vi "Initialise User login and application data.vi"(7 "mains application path":path, 8 "error in":errorcluster, 9 "Revision number":string, 10 "Strings []":string[](array[string]), 11 "Initialise cluster":T3={"wait value"=0.0, "Power supply"="COM1", "DMM"="COM1", "Arduino"="", "RS232 COM5"="", "RELAY BOARD"="COM1", "test sequence"=enum."Update Display", "Data folder path"=path "", "user account"="", "test sequence file name"="", "UI"=[], "DI"=[], "Skip test?"=[FALSE, FALSE, FALSE, FALSE, FALSE, FALSE, FALSE, FALSE, FALSE, FALSE, FALSE, FALSE, FALSE, FALSE, FALSE, FALSE, FALSE, FALSE, FALSE, FALSE, FALSE, FALSE, FALSE, FALSE, FALSE, FALSE, FALSE, FALSE, FALSE, FALSE, FALSE, FALSE], "Barcode"="", "DMM measuring state"=2, "T1"=[], "MCListbox Ref_in"=refnum, "RS232 COM6"="COM1", "mains application path"=path "", "sequence step #"=0, "Screening?"=FALSE, "Result?"=FALSE} {"DMM measuring state" items=["Voltage DC", "Voltage AC", "Current DC", "Current AC", "Resistance", "4-wire Resistance", "Diode", "Capacitance", "Temperature", "Continuity", "Frequency", "Period", "Voltage Ratio", "Voltage", "Current", "None"]; "DI"."Lower limit" format="%#_7f"}) -> (0 "error out":errorcluster, 1 "User name":i32 caption="Name(min 4 chars)", 2 "T1":string[][](array[string]), 3 "output cluster":T3={"wait value"=0.0, "Power supply"="COM1", "DMM"="COM1", "Arduino"="", "RS232 COM5"="", "RELAY BOARD"="COM1", "test sequence"=enum."Update Display", "Data folder path"=path "", "user account"="", "test sequence file name"="", "UI"=[], "DI"=[], "Skip test?"=[FALSE, FALSE, FALSE, FALSE, FALSE, FALSE, FALSE, FALSE, FALSE, FALSE, FALSE, FALSE, FALSE, FALSE, FALSE, FALSE, FALSE, FALSE, FALSE, FALSE, FALSE, FALSE, FALSE, FALSE, FALSE, FALSE, FALSE, FALSE, FALSE, FALSE, FALSE, FALSE], "Barcode"="", "DMM measuring state"=2, "T1"=[], "MCListbox Ref_in"=refnum, "RS232 COM6"="COM1", "mains application path"=path "", "sequence step #"=0, "Screening?"=FALSE, "Result?"=FALSE} {"DMM measuring state" items=["Voltage DC", "Voltage AC", "Current DC", "Current AC", "Resistance", "4-wire Resistance", "Diode", "Capacitance", "Temperature", "Continuity", "Frequency", "Period", "Voltage Ratio", "Voltage", "Current", "None"]; "DI"."Lower limit" format="%#_7f"}, 4 "Stop App?":bool, 5 "Varient&temp":T2, 6 "selected account name":string)   [LabVIEW 2021]
uses:
  controls/initialise cluster.ctl
  controls/developer_test sequence.ctl
  controls/test step description.ctl
  controls/test type selection.ctl
  controls/comparison selection.ctl
  controls/DMM measuring state.ctl
  controls/Control 1.ctl
  <vilib>/Utility/file.llb/Write Delimited Spreadsheet (string).vi
  <vilib>/Utility/file.llb/Read Delimited Spreadsheet (string).vi
panel:
  out "Data folder path":path
  out "test sequence file name":string
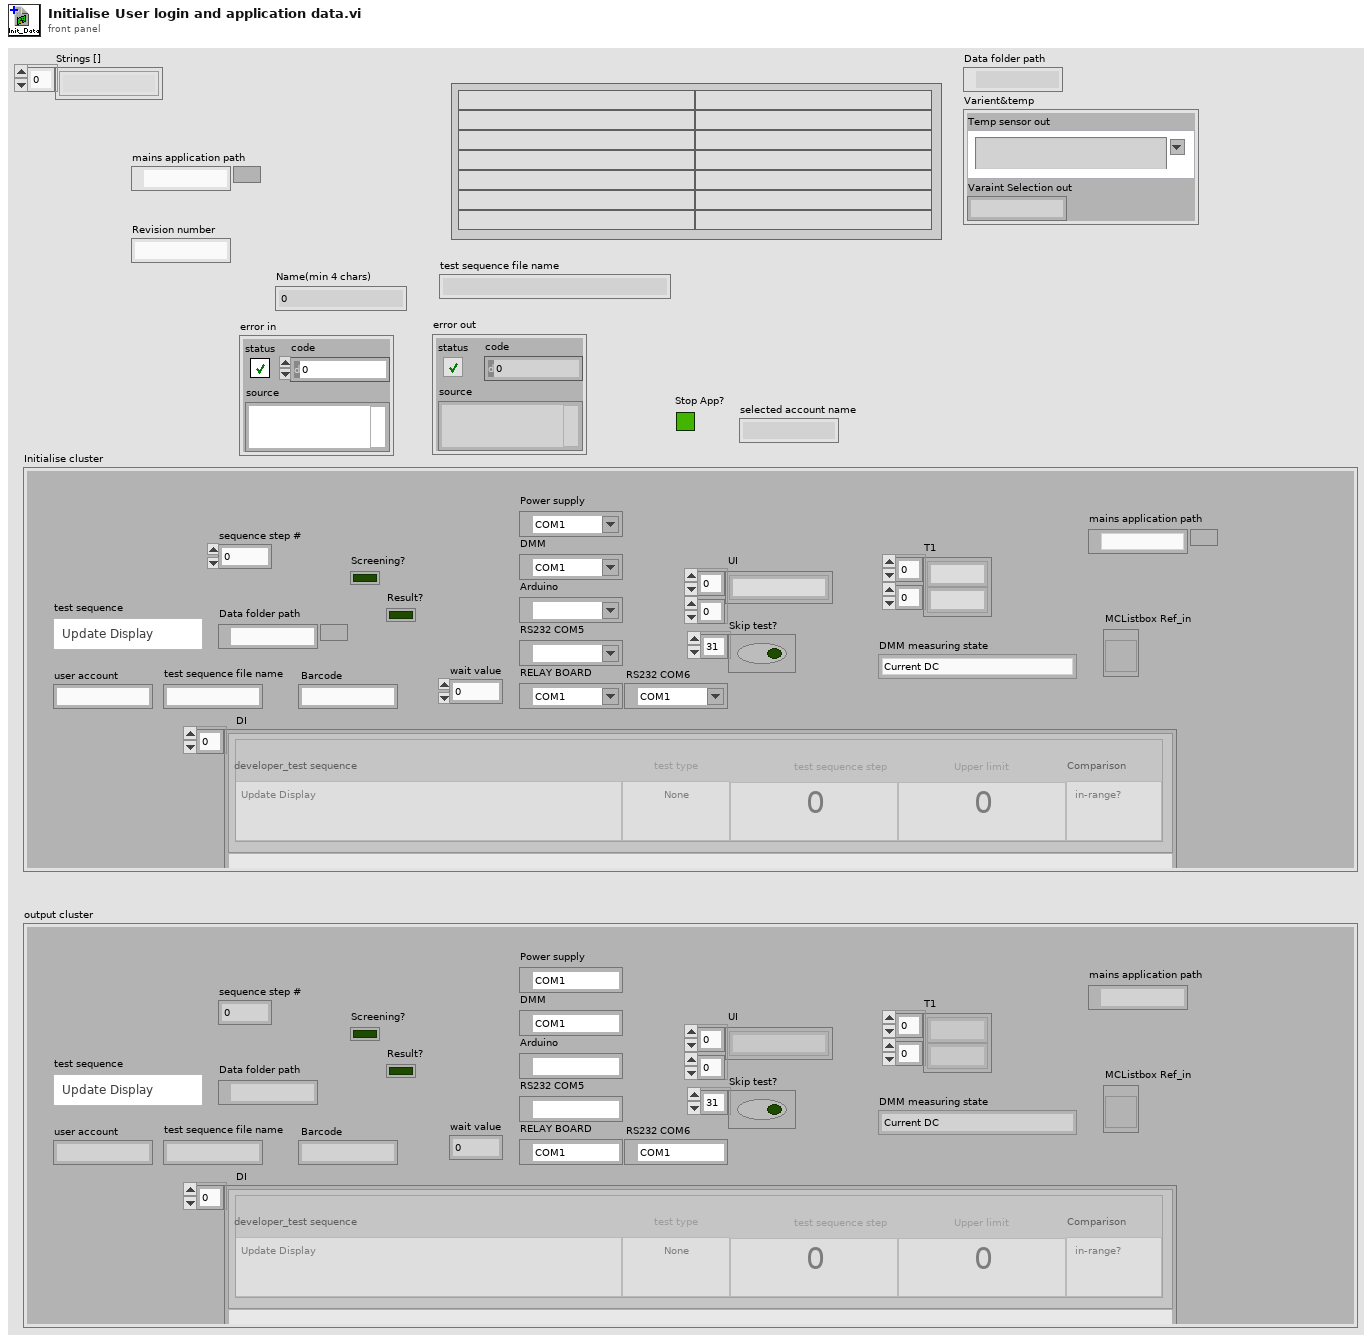
[diagram p1: front panel]
types:
  T1 = typedef "Control 1.ctl" = string
  T2 = cluster{"Temp sensor out":T1, "Varaint Selection out":string}
  T3 = typedef "initialise cluster.ctl" = cluster{"wait value":dbl, "Power supply":refnum<visa-resource-name>, "DMM":refnum<visa-resource-name>, "Arduino":refnum<visa-resource-name>, "RS232 COM5":refnum<visa-resource-name>, "RELAY BOARD":refnum<visa-resource-name>, "test sequence":T4, "Data folder path":path, "user account":string, "test sequence file name":string, "UI":string[][], "DI":T5[], "Skip test?":bool[], "Barcode":string, "DMM measuring state":T8, "T1":string[][], "MCListbox Ref_in":refnum<vi>, "RS232 COM6":refnum<visa-resource-name>, "mains application path":path, "sequence step #":u32, "Screening?":bool, "Result?":bool}
  T4 = typedef "developer_test sequence.ctl" = enum16{"Update Display", "User Login", "Admin", "Initialise", "Init Devices", "Idle State", "test steup", "Abort", "Start Display Board Auto Testing", "Scan Barcode", "Checking TEMP at Thermistor 1", "Checking TEMP at Thermistor 2", "Checking TEMP at Thermistor 3", "Checking TEMP at Thermistor 4 (Ambient)", "Voltage Health Check", "Hillpot connector check", "INSULATION Resistance test (Baseplate to Negative)", "INSULATION Resistance test (Baseplate to Positive)", "Voltage helath check before weld resistance", "Current contactor check", "WELD Resistance Test", "Stop Display Board Auto Testing", "All Pass", "Fail", "Report", "Error", "Confirm Quit", "Exit"}
  T5 = typedef "test step description.ctl" = cluster{"test type":T6, "developer_test sequence":T4, "Lower limit":dbl, "Upper limit":dbl, "Comparison":T7}
  T6 = typedef "test type selection.ctl" = enum16{"None", "Voltage", "Voltage?", "Current", "Current?", "Output", "Program"}
  T7 = typedef "comparison selection.ctl" = enum16{"None", "in-range?", "less than?", "greater than?", "equal to?", "not equal to?", "less or equal to?", "greater or equal to?"}
  T8 = typedef "DMM measuring state.ctl" = u16
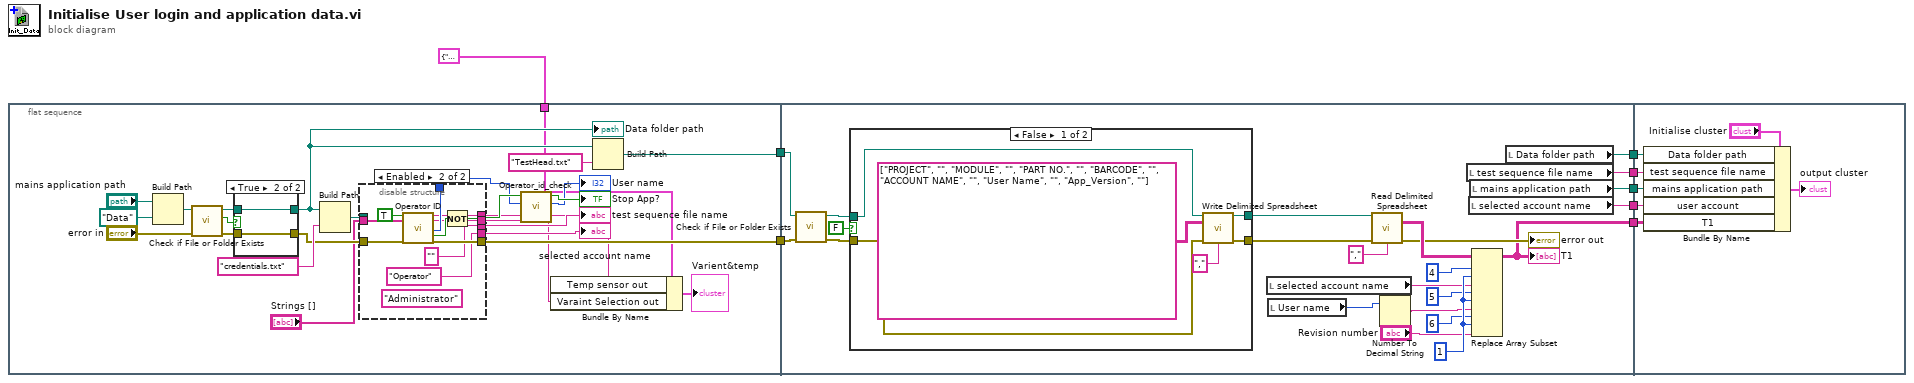
[diagram p0: block diagram]
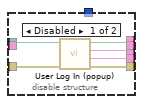
[diagram p2: hidden frame]
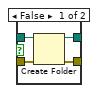
[diagram p3: hidden frame]
diagram:
  n1 = flat-sequence {
    tunnel: [w23] -> w8
    tunnel: [w19] -> w4
    tunnel: T2 {"Temp sensor out"="", "Varaint Selection out"=""} -> [w13]
    tunnel: w8 -> [w66]
    tunnel: [w71] -> w7
    tunnel: [w65] -> w6
    tunnel: [w64] -> w5
    tunnel: w4 -> [w63]
    tunnel: [w62] -> w3
    tunnel: [w61] -> w2
    tunnel: w7 -> [w93]
    tunnel: w6 -> [w91]
    tunnel: w5 -> [w90]
    tunnel: w3 -> [w89]
    tunnel: w2 -> [w88]
    frame #0 {
      n2 = Build Path(base path="mains application path", name or relative path=path "Data") -> (appended path=w26:path)
      n3 = call <vilib>:"Check if File or Folder Exists.vi"("error in (no error)"="error in", "path"=w26) -> ("error out"=w30:errorcluster, "file or folder exists?"=w32:bool, "dup path"=w31:path)  [unwired: 7 in]
      n4 = case shown="True" w32 {
        tunnel: w31 -> [w54 w56]
        tunnel: w30 -> [w53 w55]
        tunnel: [w52 w56] -> w18
        tunnel: [w51 w55] -> w27
        frame False {
          n5 = Create Folder(path (use dialog)=w54, error in=w53) -> (created path=w52:path, error out=w51:errorcluster)  [unwired: 1 in, 1 out]
        }
        frame True {
        }
      }
      "Data folder path" <- w18
      n6 = Build Path(base path=w18, name or relative path="credentials.txt") -> (appended path=w28:path)
      n7 = disable-structure shown="Enabled" {
        disable-tunnel: w28 -> [w39 _]
        disable-tunnel: w27 -> [w38 w49]
        disable-tunnel: [w37 w44] -> w16
        disable-tunnel: [w36 "" ("test sequence file name")] -> w24
        disable-tunnel: [_ w47] -> w15
        disable-tunnel: [w35 w48] -> w23
        disable-tunnel: [w34 "Operator" ("selected account name")] -> w21
        disable-tunnel: [_ w42] -> w12
        disable-tunnel: [_ w41] -> w11
        disable-tunnel: "Strings []" -> [_ w40]
        frame Disabled {
          n8 = call "User Log In (popup).vi"("error in (no error)"=w38, "Path"=w39) -> ("error out"=w35:errorcluster, "selected account name"=w34:string, "test sequence file name"=w36:string, "Stop App?"=w37:bool)  [unwired: 5 in, 1 out]
        }
        frame Enabled {
          (unwired) "Administrator" ("selected account name")
          n9 = call "Operator ID.vi"("Enable"=TRUE, "Strings []"=w40, "error in (no error)"=w49) -> ("Temp sensor out"=w42:T1, "Varaint Selection out"=w41:string, "Operator ID"=w47:i32, "OK"=w43:bool, "error out"=w48:errorcluster)  [unwired: 12 in]
          n10 = Not(x=w43) -> (.not. x?=w44:bool)
        }
      }
      "test sequence file name" <- w24
      "selected account name" <- w21
      n11 = call "Operator_id_check.vi"("Numeric 2"=w15, "in"=w16) -> ("Numeric"=→"User name":i32, "out"=→"Stop App?":bool)  [unwired: 8 in]
      n12 = Bundle By Name(cluster=w13, "Temp sensor out"=w12, "Varaint Selection out"=w11) -> (→"Varient&temp":T2)
      n13 = Build Path(base path=w18, name or relative path="TestHead.txt") -> (appended path=w19:path)
    }
    frame #1 {
      w76 = 1 ("disabled index (col)")
      n14 = call <vilib>:"Check if File or Folder Exists.vi"("error in (no error)"=w66, "path"=w63) -> ("error out"=w70:errorcluster, "dup path"=w69:path)  [unwired: 7 in, 1 out]
      n15 = case shown="False" FALSE {
        tunnel: w69 -> [w85 w87]
        tunnel: w70 -> [w83 w86]
        tunnel: [w82 w87] -> w68
        tunnel: [w81 w86] -> w67
        frame False {
          n16 = call-poly <vilib>:"Write Delimited Spreadsheet.vi"("file path (dialog if empty)"=w85, "2D data"=string[][] [["PROJECT", ""], ["MODULE", ""], ["PART NO.", ""], ["BARCODE", ""], ["ACCOUNT NAME", ""], ["User Name", ""], ["App_Version", ""]], "error in (no error)"=w83, "delimiter (\\t)"="," ("delimiter (\\t)")) -> ("new file path (Not A Path if cancelled)"=w82:path, "error out"=w81:errorcluster)  [unwired: 10 in]
        }
        frame True {
        }
      }
      n17 = local read "selected account name"() -> (w72:string)
      n18 = local read "User name"() -> (w58:i32)
      n19 = call-poly <vilib>:"Read Delimited Spreadsheet.vi"("file path (dialog if empty)"=w68, "error in (no error)"=w67, "delimiter (\\t)"=",") -> ("all rows"=w79:string[][], "error out"=→"error out":errorcluster)  [unwired: 7 in, 4 out]
      n20 = Number To Decimal String(number=w58) -> (decimal integer string=w57:string)  [unwired: 1 in]
      n21 = local read "test sequence file name"() -> (w62:string)
      n22 = local read "selected account name"() -> (w65:string)
      n23 = local read "mains application path"() -> (w64:path)
      n24 = Replace Array Subset(array=w79, new element #1=w72, index (row) #1=4 ("index (row)"), index (col) #1=w76, new element #2=w57, index (row) #2=5 ("disabled index (row)"), index (col) #2=w76, new element #3="Revision number", index (row) #3=6 ("disabled index (row)"), index (col) #3=w76) -> (w71:string[][])
      "T1" <- w71
      n25 = local read "Data folder path"() -> (w61:path)
    }
    frame #2 {
      n26 = Bundle By Name(cluster="Initialise cluster", "Data folder path"=w88, "test sequence file name"=w89, "mains application path"=w90, "user account"=w91, "T1"=w93) -> (→"output cluster":T3)
    }
  }
